vi "Write.vi"(8 "error in (no error)":errorcluster, 9 "timeout ms (5000)":i32=5000, 10 "Bytes to write":u8[](array[numeric]), 11 "dotNET TCP Socket in":refnum<class "dotNET TCP Socket.lvclass">) -> (0 "error out":errorcluster, 2 "bytes written":i32, 3 "dotNET TCP Socket out":refnum<class "dotNET TCP Socket.lvclass">)   [LabVIEW 2013, in "dotNET SSL Socket.lvlib" / "dotNET TCP Socket.lvclass"]
doc: "Writes data to the socket.\nWebSockets 2.0.0.32\nSam Sharp - MediaMongrels Ltd\nCopyright (c) 2019, MediaMongrels Ltd"
uses:
  dotNET TCP Socket.lvclass
  dotNET TCP Socket.lvclass/dotNET TCP Socket.ctl
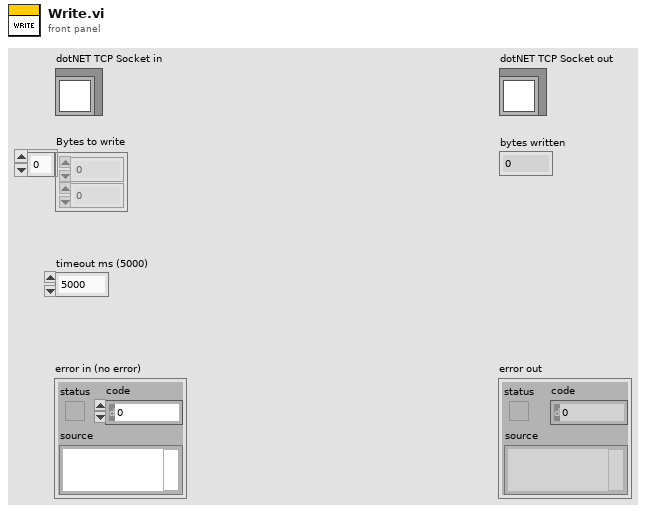
[diagram p1: front panel]
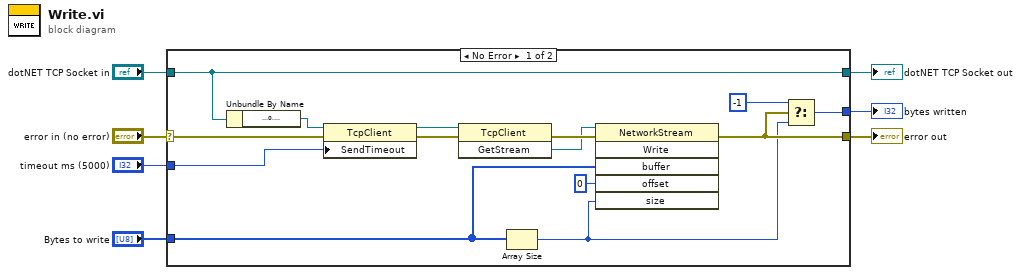
[diagram p0: block diagram]
diagram:
  n1 = case shown="No Error" "error in (no error)" {
    selector: "error in (no error)" -> [w13 w23]
    tunnel: "dotNET TCP Socket in" -> [w12 w22]
    tunnel: "timeout ms (5000)" -> [w19 _]
    tunnel: "Bytes to write" -> [w10 _]
    tunnel: [w15 w23] -> w4
    tunnel: [w14 _] -> w3
    tunnel: [w12 w22] -> w1
    frame No Error {
      n2 = Unbundle By Name(w12) -> ("TcpClient"=w20:refnum<k24>)
      n3 = property class="TcpClient"(reference=w20, error in=w13, "SendTimeout"=w19) -> (reference out=w18:refnum<k24>, error out=w17:errorcluster)
      n4 = invoke class="TcpClient" method="GetStream"(reference=w18, error in=w17) -> (error out=w16:errorcluster, "GetStream"=w11:refnum<k24>)  [unwired: 1 in, 1 out]
      n5 = Array Size(array=w10) -> (size(s)=w8:i32)
      n6 = invoke class="NetworkStream" method="Write"(reference=w11, error in=w16, "buffer"=w10, "offset"=0, "size"=w8) -> (error out=w15:errorcluster)  [unwired: 1 in, 5 out]
      n7 = Select(t=-1, s=w15, f=w8) -> (s? t:f=w14:i32)
    }
    frame Error {
    }
  }
  "error out" <- w4
  "dotNET TCP Socket out" <- w1
  "bytes written" <- w3
